vi "Node ID Map.vi"(8 "error in (no error)":errorcluster, 11 "Cluster in":refnum<class "Cluster.lvclass">) -> (0 "error out":errorcluster, 2 "Node ID Map":map{string, u32}(c390), 3 "Cluster out":refnum<class "Cluster.lvclass">)   [LabVIEW 2020, in "VolatusConfig.lvlib" / "Cluster.lvclass"]
uses:
  Cluster.lvclass
  Cluster.lvclass/Cluster.ctl
  VolatusConfigElement/VolatusConfigElement.lvclass
  VolatusConfig.lvlib
  Meta Type.ctl
  Node/Node.lvclass
  C:/dev/lv20CE/relink/lv-volatus/VolatusConfig/VolatusConfigElement/VolatusConfigElement.lvclass
  C:/dev/lv20CE/relink/lv-volatus/VolatusConfig/Cluster/Cluster.lvclass
  C:/dev/lv20CE/relink/lv-volatus/VolatusConfig/Node/Node.lvclass
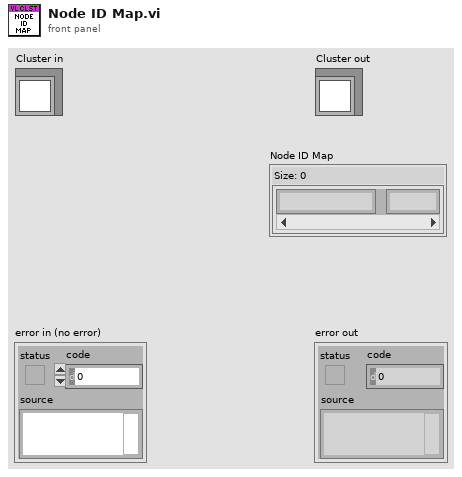
[diagram p1: front panel]
types:
  T1 = typedef "VolatusConfig.lvlib/Meta Type.ctl" = enum16{"UNKNOWN", "VL_System", "VL_Cluster", "VL_Node", "VL_Task", "VL_Group", "VL_Channel", "VL_Task_List", "VL_Scaling", "VL_Sensor", "VL_Sensor_List", "VL_Scale"}
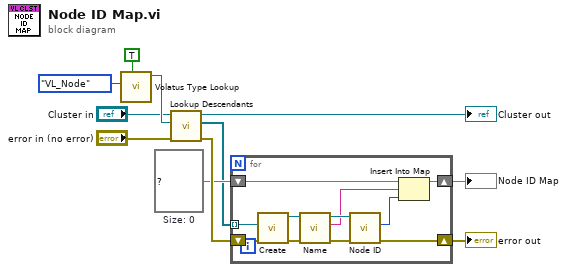
[diagram p0: block diagram]
diagram:
  w7 = map{string, u32} {}  # Size: 0
  n1 = call "Volatus Type Lookup.vi"("Don't Recurse Past Match (F)"=TRUE, "Meta Type"=Meta_Type."VL_Node") -> ("Config Lookup out"=w9:refnum<class "Config Lookup.lvclass">)  [unwired: 8 in, 1 out]
  n2 = call "Lookup Descendants.vi"("error in (no error)"="error in (no error)", "Lookup"=w9, "VolatusConfigElement in"="Cluster in") -> ("error out"=w11:errorcluster, "Descendants"=w6:refnum<class "Config Element.lvclass">[], "VolatusConfigElement out"=→"Cluster out":refnum<class "Cluster.lvclass">)  [unwired: 6 in]
  n3 = for {
    shift-right: [w12] -> w1
    shift-left: w7 -> [w16]
    tunnel: w6 -> [w22] mode=indexing
    shift-right: [w13] -> w2
    shift-left: w11 -> [w20]
    n4 = call "Create.vi"("error in (no error)"=w20, "Element"=w22) -> ("error out"=w19:errorcluster, "Node out"=w21:refnum<class "Node.lvclass">)  [unwired: 8 in]
    n5 = call "Name.vi"("error in (no error)"=w19, "VolatusConfigElement in"=w21) -> ("error out"=w17:errorcluster, "Name"=w14:string, "VolatusConfigElement out"=w18:refnum<class "Node.lvclass">)  [unwired: 7 in]
    n6 = call "Node ID.vi"("error in (no error)"=w17, "Node in"=w18) -> ("error out"=w13:errorcluster, "Node ID"=w15:u32)  [unwired: 7 in, 1 out]
    n7 = Insert Into Map(map in=w16, key=w14, value=w15) -> (map out=w12:map{string, u32})  [unwired: 2 out]
  }
  "error out" <- w2
  "Node ID Map" <- w1
